vi "Lint Library.vi"(8 "Error In":errorcluster, 10 "Results In":T1[](array[typedef]), 11 "Project Item In":refnum<vi>) -> (0 "Error Out":errorcluster, 2 "Results Out":T1[](array[typedef]), 3 "Project Item Out":refnum<vi>)   [LabVIEW 2018, in "Scripts.lvlib"]
uses:
  Scripts.lvlib
  Project Item Lint Result.ctl
  VI Control Lint Result.ctl
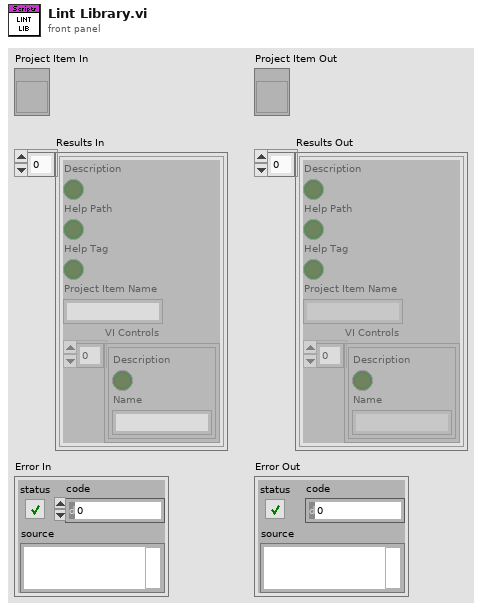
[diagram p1: front panel]
types:
  T1 = typedef "Scripts.lvlib/Project Item Lint Result.ctl" = cluster{"Description":bool, "Help Path":bool, "Help Tag":bool, "Project Item Name":string, "VI Controls":T2[]}
  T2 = typedef "Scripts.lvlib/VI Control Lint Result.ctl" = cluster{"Description":bool, "Name":string}
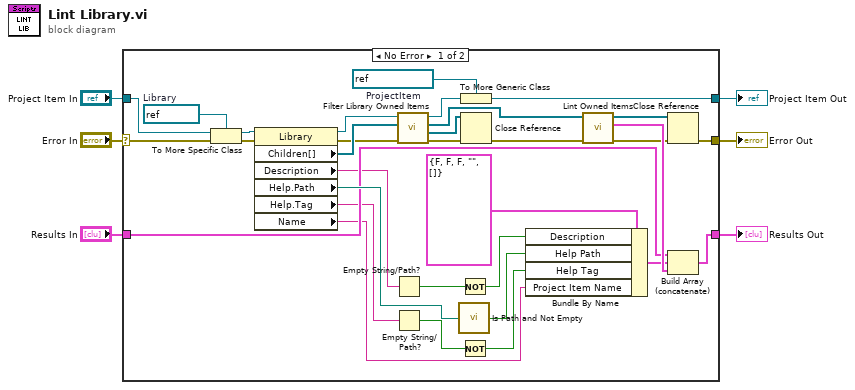
[diagram p0: block diagram]
diagram:
  n1 = case shown="No Error" "Error In" {
    selector: "Error In" -> [w7 w41]
    tunnel: [w36 w39] -> w6
    tunnel: "Results In" -> [w33 w39]
    tunnel: [w19 w40] -> w4
    tunnel: "Project Item In" -> [w16 w40]
    tunnel: [w15 w41] -> w2
    frame No Error {
      w20 = refnum<vi> refnum  # ProjectItem
      w18 = refnum<vi> refnum  # Library
      n2 = To More Specific Class(target class=w18, reference=w16, error in=w7) -> (specific class reference=w17:refnum<vi>, error out=w22:errorcluster)
      n3 = property class="Library"(reference=w17, error in=w22) -> (reference out=w21:refnum<vi>, error out=w23:errorcluster, "Children[]"=w32:refnum<vi>[], "Description"=w31:string, "Help.Path"=w37:path, "Help.Tag"=w27:string, "Name"=w30:string)
      n4 = Empty String/Path?(string/path=w31) -> (empty?=w25:bool)
      n5 = Empty String/Path?(string/path=w27) -> (empty?=w26:bool)
      n6 = call "Filter Library Owned Items.vi"("Error In"=w23, "Children[]"=w32, "Library Project Item In"=w21) -> ("Error Out"=w10:errorcluster, "Private Owned Items"=w12:refnum<vi>[], "Non-Private Owned Items"=w9:refnum<vi>[], "Library Project Item Out"=w8:refnum<vi>)  [unwired: 5 in]
      n7 = call <vilib>:"Is Path and Not Empty.vi"("path"=w37) -> ("Is Path and Not Empty?"=w38:bool)  [unwired: 4 in]
      n8 = Not(x=w25) -> (.not. x?=w28:bool)
      n9 = Not(x=w26) -> (.not. x?=w29:bool)
      n10 = To More Generic Class(target class=w20, reference=w8) -> (generic class reference=w19:refnum<vi>)
      n11 = Close Reference(reference=w12, error in (no error)=w10) -> (error out=w11:errorcluster)
      n12 = Bundle By Name(cluster=T1 {"Description"=FALSE, "Help Path"=FALSE, "Help Tag"=FALSE, "Project Item Name"="", "VI Controls"=[]} ("Lint Result"), "Description"=w28, "Help Path"=w38, "Help Tag"=w29, "Project Item Name"=w30) -> (w34:T1)
      n13 = call "Lint Owned Items.vi"("Error In"=w11, "Owned Items In"=w9) -> ("Error Out"=w14:errorcluster, "Results"=w35:T1[], "Owned Items Out"=w13:refnum<vi>[])  [unwired: 7 in]
      n14 = Close Reference(reference=w13, error in (no error)=w14) -> (error out=w15:errorcluster)
      n15 = Build Array (concatenate)(w33, w34, w35) -> (w36:T1[])
    }
    frame Error {
    }
  }
  "Results Out" <- w6
  "Project Item Out" <- w4
  "Error Out" <- w2
